vi "Read.vi"(8 "error in (no error)":errorcluster, 9 "Timeout S (0)":dbl, 10 "Bytes to Read (0)":i32, 11 "DeployResource in":refnum<class "Resource.lvclass">) -> (0 "error out":errorcluster, 1 "Bytes Read":i32, 2 "Data":string, 3 "DeployResource out":refnum<class "Resource.lvclass">)   [LabVIEW 2020, in "PicoG-Core.lvlib" / "Resource.lvclass"]
doc: "<b>Bytes to Read</b>:\n -1 to read as many bytes as possible until timeout\n 0 to return current bytes available immediately, ignoring timeout.\n >0 to wait for number of bytes until timeout"
uses:
  Resource.lvclass
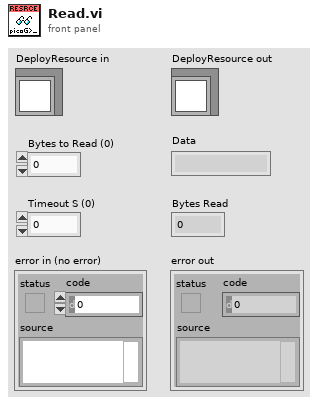
[diagram p1: front panel]
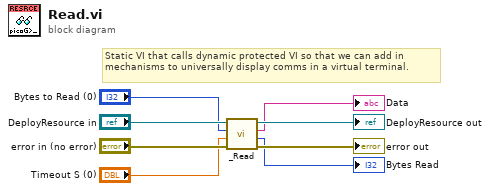
[diagram p0: block diagram]
diagram:
  # "Static VI that calls dynamic protected VI so that we can add in mechanisms to universally display comms in a virtual terminal."
  n1 = call-dynamic "_Read.vi"("error in (no error)"="error in (no error)", "Timeout S (0)"="Timeout S (0)", "Bytes to Read (0)"="Bytes to Read (0)", "DeployResource in"="DeployResource in") -> ("error out"=→"error out":errorcluster, "Bytes Read"=→"Bytes Read":i32, "Data"=→"Data":string, "DeployResource out"=→"DeployResource out":refnum<class "Resource.lvclass">)  [unwired: 4 in]
